vi "Determine Message Type.vi"(8 "error in":errorcluster, 10 "Item Refnum":refnum<vi>) -> (0 "error out":errorcluster, 2 "Enum":T1(ring))   [LabVIEW 2020, in "Message Rescripter.lvlib"]
uses:
  Message Rescripter.lvlib
  MessageMakerProvider/_Message Maker/Message Maker.lvlib
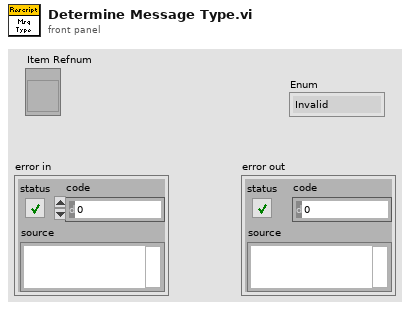
[diagram p1: front panel]
types:
  T1 = enum16{"Invalid", "Abstract", "Concrete", "Standard"}
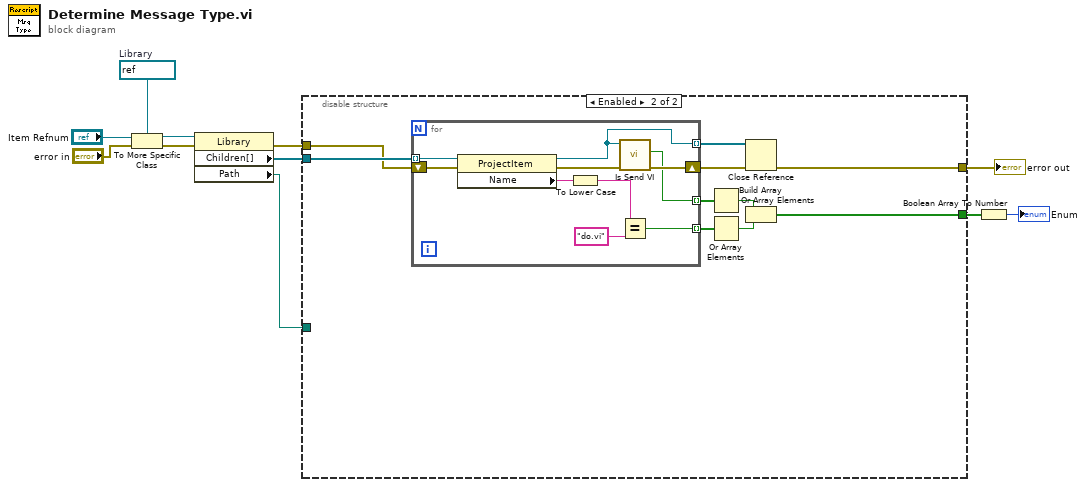
[diagram p0: block diagram]
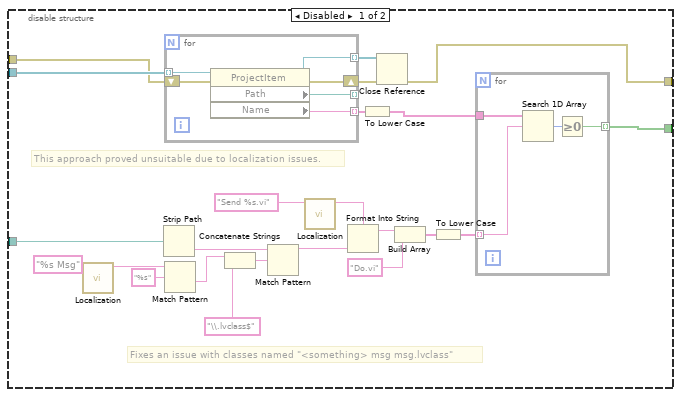
[diagram p2: hidden frame]
diagram:
  w11 = refnum<vi> refnum  # Library
  n1 = To More Specific Class(target class=w11, reference="Item Refnum", error in="error in") -> (specific class reference=w9:refnum<vi>, error out=w10:errorcluster)
  n2 = property class="Library"(reference=w9, error in=w10) -> (error out=w4:errorcluster, "Children[]"=w7:refnum<vi>[], "Path"=w2:path)  [unwired: 1 out]
  n3 = disable-structure shown="Enabled" {
    disable-tunnel: w7 -> [w34 w52]
    disable-tunnel: [w30 w46] -> w6
    disable-tunnel: w4 -> [w29 w51]
    disable-tunnel: w2 -> [w28 _]
    disable-tunnel: [w27 w45] -> w1
    frame Disabled {
      # "This approach proved unsuitable due to localization issues."
      # "Fixes an issue with classes named \"<something> msg msg.lvclass\""
      n4 = call "Localization.vi"("Unlocalized"="%s Msg" ("Name of new Message Class (without .lvclass file extension)")) -> ("Localized"=w23:string)  [unwired: 10 in]
      n5 = Strip Path(path=w28) -> (name=w20:string)  [unwired: 1 out]
      n6 = for {
        tunnel: w34 -> [w44] mode=indexing
        tunnel: [w40] -> w31 mode=indexing
        shift-right: [w42] -> w33
        shift-left: w29 -> [w43]
        tunnel: [w41] -> w32 mode=indexing
        tunnel: [w39] -> _ mode=indexing
        n7 = property class="ProjectItem"(reference=w44, error in=w43) -> (reference out=w41:refnum<vi>, error out=w42:errorcluster, "Path"=w39:path, "Name"=w40:string)
      }
      n8 = Match Pattern(string=w23, regular expression="%s") -> (after substring=w21:string)  [unwired: 1 in, 3 out]
      n9 = Concatenate Strings(w21, "\\.lvclass$" ("string")) -> (w15:string)
      n10 = Match Pattern(string=w20, regular expression=w15) -> (before substring=w13:string)  [unwired: 1 in, 3 out]
      n11 = call "Localization.vi"("Unlocalized"="Send %s.vi") -> ("Localized"=w26:string)  [unwired: 10 in]
      n12 = Format Into String(format string=w26, w13) -> (resulting string=w19:string)  [unwired: 2 in, 1 out]
      n13 = To Lower Case(string=w31) -> (all lower case string=w12:string[])
      n14 = Close Reference(reference=w32, error in (no error)=w33) -> (error out=w27:errorcluster)
      n15 = Build Array(w19, "Do.vi" ("element")) -> (w17:string[])
      n16 = To Lower Case(string=w17) -> (all lower case string=w16:string[])
      n17 = for {
        tunnel: w12 -> [w38]
        tunnel: w16 -> [w37] mode=indexing
        tunnel: [w35] -> w30 mode=indexing
        n18 = Search 1D Array(1D array=w38, element=w37) -> (index of element=w36:i32)  [unwired: 1 in]
        n19 = Greater Or Equal To 0?(x=w36) -> (x >= 0?=w35:bool)
      }
    }
    frame Enabled {
      n20 = for {
        tunnel: w52 -> [w64] mode=indexing
        shift-right: [w61] -> w54
        shift-left: w51 -> [w63]
        tunnel: [w57] -> w53 mode=indexing
        tunnel: [w56] -> w49 mode=indexing
        tunnel: [w55] -> w50 mode=indexing
        n21 = property class="ProjectItem"(reference=w64, error in=w63) -> (reference out=w57:refnum<vi>, error out=w62:errorcluster, "Name"=w59:string)
        n22 = To Lower Case(string=w59) -> (all lower case string=w58:string)
        n23 = call "Is Send VI.vi"("error in (no error)"=w62, "ProjectItem in"=w57) -> ("error out"=w61:errorcluster, "Is Send VI?"=w55:bool)  [unwired: 7 in, 1 out]
        n24 = Equal?(x=w58, y="do.vi" ("element")) -> (x = y?=w56:bool)
      }
      n25 = Or Array Elements(Boolean array=w50) -> (logical OR=w48:bool)
      n26 = Or Array Elements(Boolean array=w49) -> (logical OR=w47:bool)
      n27 = Close Reference(reference=w53, error in (no error)=w54) -> (error out=w45:errorcluster)
      n28 = Build Array(w48, w47) -> (w46:bool[])
    }
  }
  "error out" <- w1
  n29 = Boolean Array To Number(Boolean array=w6) -> (number=→"Enum":u32)
